vi "Run_Core.vi"(0 "Message Popup in":refnum<class "print screen.lvclass">, 11 "error in (no error)":errorcluster) -> (4 "Message Popup out":refnum<class "print screen.lvclass">, 6 "Return":variant, 15 "error out":errorcluster)   [LabVIEW 2016, in "print screen.lvclass"]
uses:
  print screen.lvclass
  D:/TOOLS/Funtion_Lists/source code/LSL components/functions/functionsbase/functionbase.lvclass
  functionsbase/functionbase.lvclass/functionbase.ctl
  print screen.lvclass/print screen.ctl
  functionsbase/properties/Read Output Terminal.vi
  functionsbase/properties/Read Smart Syntax Representation.vi
  output terminal/Base/Output Terminal.lvclass
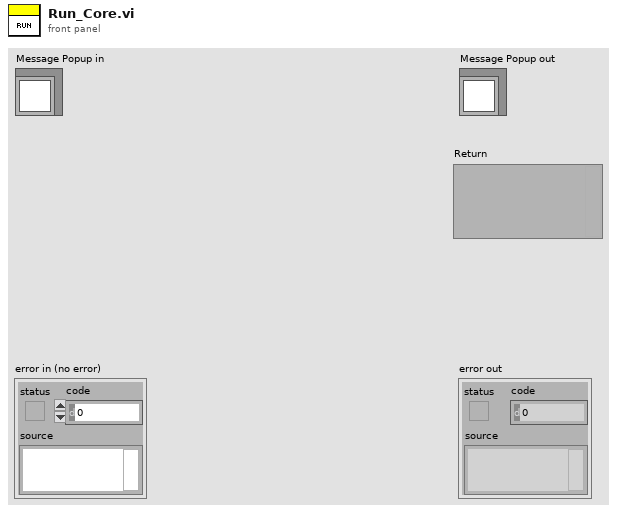
[diagram p1: front panel]
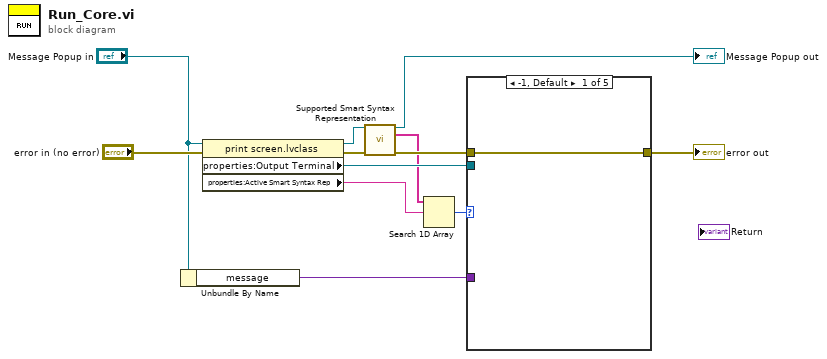
[diagram p0: block diagram]
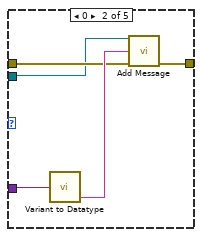
[diagram p2: hidden frame]
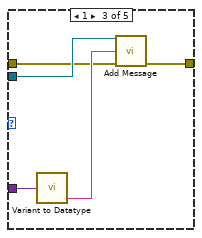
[diagram p3: hidden frame]
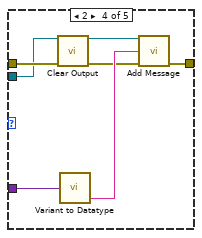
[diagram p4: hidden frame]
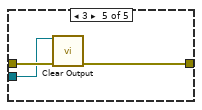
[diagram p5: hidden frame]
diagram:
  n1 = Unbundle By Name("Message Popup in") -> ("message"=w8:variant)
  n2 = property class="print screen.lvclass"(reference="Message Popup in", error in="error in (no error)") -> (reference out=w4:refnum<class "print screen.lvclass">, error out=w7:errorcluster, "properties:Output Terminal"=w9:refnum<class "Output Terminal.lvclass">, "properties:Active Smart Syntax Rep"=w2:string)
  n3 = call-dynamic "Supported Smart Syntax Representation.vi"("Message Popup in"=w4, "error in (no error)"=w7) -> ("Message Popup out"=→"Message Popup out":refnum<class "print screen.lvclass">, "Smart Syntax Representation List"=w5:string[], "error out"=w6:errorcluster)  [unwired: 11 in]
  n4 = Search 1D Array(1D array=w5, element=w2) -> (index of element=w1:i32)  [unwired: 1 in]
  n5 = case shown="-1, Default" w1 {
    tunnel: [w13 w16 w23 w30 w32] -> w10
    tunnel: w9 -> [_ w15 w22 w25 w31]
    tunnel: w8 -> [_ w14 w21 w29 _]
    tunnel: w6 -> [w13 w17 w19 w27 w33]
    frame -1, Default {
    }
    frame 0 {
      n6 = call "Variant to Datatype.vi"("Variant"=w14) -> ("Value"=w18:string)  [unwired: 2 in, 2 out]
      n7 = call-dynamic "Add Message.vi"("Output Terminal in"=w15, "Message"=w18, "error in (no error)"=w17) -> ("error out"=w16:errorcluster)  [unwired: 11 in, 1 out]
    }
    frame 1 {
      n8 = call "Variant to Datatype.vi"("Variant"=w21) -> ("Value"=w20:string)  [unwired: 2 in, 2 out]
      n9 = call-dynamic "Add Message.vi"("Output Terminal in"=w22, "Message"=w20, "error in (no error)"=w19) -> ("error out"=w23:errorcluster)  [unwired: 11 in, 1 out]
    }
    frame 2 {
      n10 = call-dynamic "Clear Output.vi"("Output Terminal in"=w25, "error in (no error)"=w27) -> ("Output Terminal out"=w24:refnum<class "Output Terminal.lvclass">, "error out"=w26:errorcluster)  [unwired: 12 in]
      n11 = call "Variant to Datatype.vi"("Variant"=w29) -> ("Value"=w28:string)  [unwired: 2 in, 2 out]
      n12 = call-dynamic "Add Message.vi"("Output Terminal in"=w24, "Message"=w28, "error in (no error)"=w26) -> ("error out"=w30:errorcluster)  [unwired: 11 in, 1 out]
    }
    frame 3 {
      n13 = call-dynamic "Clear Output.vi"("Output Terminal in"=w31, "error in (no error)"=w33) -> ("error out"=w32:errorcluster)  [unwired: 12 in, 1 out]
    }
  }
  "error out" <- w10
